vi "Update Indicators.vi"(8 "error in (no error)":errorcluster, 11 "Bioreactor in":refnum<class "Bioreactor.lvclass">) -> (0 "error out":errorcluster, 3 "Bioreactor out":refnum<class "Bioreactor.lvclass">)   [LabVIEW 2013, in "Bioreactor.lvlib" / "Bioreactor.lvclass"]
uses:
  Bioreactor.lvclass
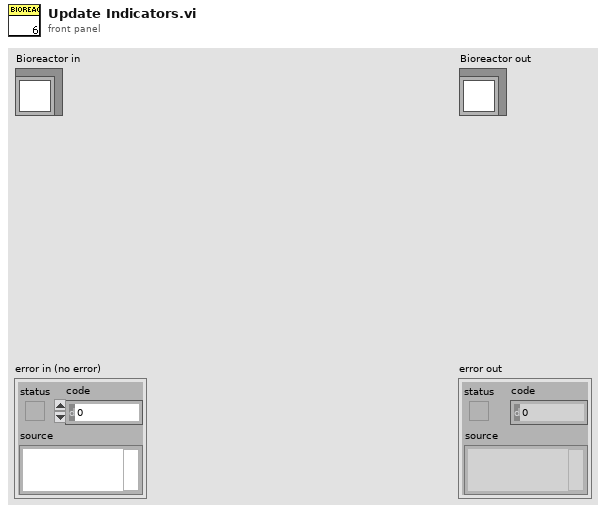
[diagram p1: front panel]
types:
  T1 = cluster{"output array":dbl[], "output array":dbl[]}
  T2 = cluster{"output array":dbl[], "output array":dbl[]}[]
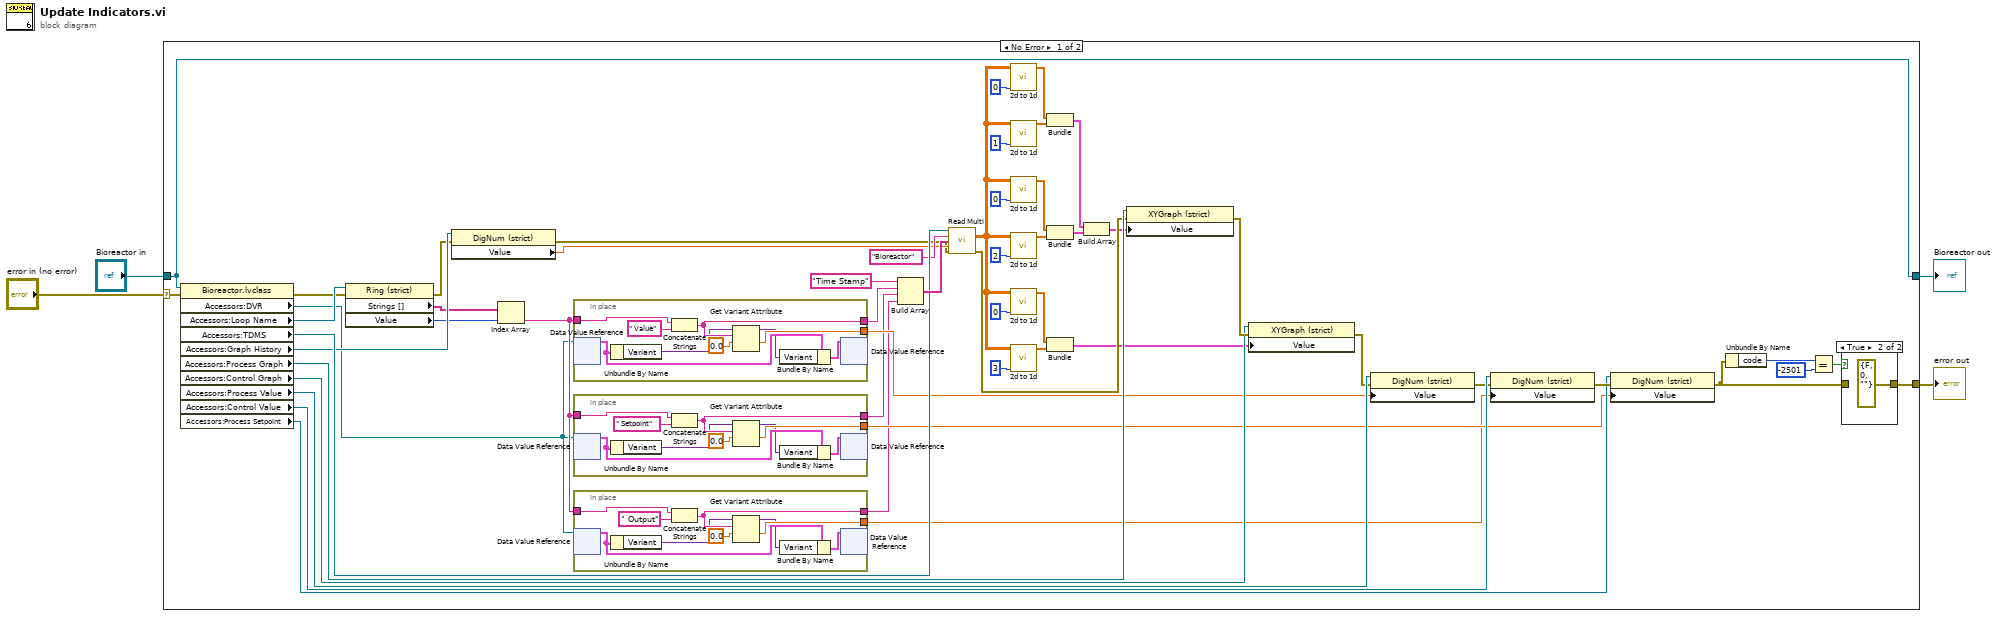
[diagram p0: block diagram]
diagram:
  n1 = case shown="No Error" "error in (no error)" {
    selector: "error in (no error)" -> [w54 w89]
    tunnel: [w18 w89] -> w3
    tunnel: [w58 w88] -> w1
    tunnel: "Bioreactor in" -> [w58 w88]
    frame No Error {
      n2 = property class="Bioreactor.lvclass"(reference=w58, error in=w54) -> (error out=w53:errorcluster, "Accessors:DVR"=w5:refnum<data-value>, "Accessors:Loop Name"=w55:refnum<vi>, "Accessors:TDMS"=w48:refnum<k34>, "Accessors:Graph History"=w37:refnum<vi>, "Accessors:Process Graph"=w35:refnum<vi>, "Accessors:Control Graph"=w36:refnum<vi>, "Accessors:Process Value"=w57:refnum<vi>, "Accessors:Control Value"=w56:refnum<vi>, "Accessors:Process Setpoint"=w50:refnum<vi>)  [unwired: 1 out]
      n3 = property class="Ring (strict)"(reference=w55, error in=w53) -> (error out=w17:errorcluster, "Strings []"=w15:string[], "Value"=w16:u16)  [unwired: 1 out]
      n4 = property class="DigNum (strict)"(reference=w37, error in=w17) -> (error out=w13:errorcluster, "Value"=w14:dbl)  [unwired: 1 out]
      n5 = Index Array(array=w15, index=w16) -> (element=w6:string)
      n6 = in-place {
        in-place-border: w6 -> [w67]
        in-place-border: [w64] -> w12
        in-place-border: [w63] -> w7
        n7 = in-place-dvr #1(w5) -> (w62:cluster{"Array":string[], "Variant":variant})  [unwired: 1 out]
        n8 = Unbundle By Name(w62) -> ("Variant"=w61:variant)
        n9 = Concatenate Strings(w67, " Value" ("string")) -> (w63:string)
        n10 = Get Variant Attribute(Variant=w61, name=w63, default value (empty Variant)=0.0 ("Value")) -> (duplicate Variant=w60:variant, value=w64:dbl)  [unwired: 1 in, 2 out]
        n11 = Bundle By Name(cluster=w62, "Variant"=w60) -> (w59:cluster{"Array":string[], "Variant":variant})
        n12 = in-place-dvr #1(w59) -> ()  [unwired: 2 out]
      }
      n13 = in-place {
        in-place-border: w6 -> [w85]
        in-place-border: [w84] -> w11
        in-place-border: [w81] -> w9
        n14 = in-place-dvr #2(w5) -> (w80:cluster{"Array":string[], "Variant":variant})  [unwired: 1 out]
        n15 = Unbundle By Name(w80) -> ("Variant"=w79:variant)
        n16 = Concatenate Strings(w85, " Setpoint" ("string")) -> (w81:string)
        n17 = Get Variant Attribute(Variant=w79, name=w81, default value (empty Variant)=0.0 ("Value")) -> (duplicate Variant=w78:variant, value=w84:dbl)  [unwired: 1 in, 2 out]
        n18 = Bundle By Name(cluster=w80, "Variant"=w78) -> (w77:cluster{"Array":string[], "Variant":variant})
        n19 = in-place-dvr #2(w77) -> ()  [unwired: 2 out]
      }
      n20 = in-place {
        in-place-border: w6 -> [w76]
        in-place-border: [w75] -> w10
        in-place-border: [w72] -> w8
        n21 = in-place-dvr #3(w5) -> (w71:cluster{"Array":string[], "Variant":variant})  [unwired: 1 out]
        n22 = Unbundle By Name(w71) -> ("Variant"=w70:variant)
        n23 = Concatenate Strings(w76, " Output" ("string")) -> (w72:string)
        n24 = Get Variant Attribute(Variant=w70, name=w72, default value (empty Variant)=0.0 ("Value")) -> (duplicate Variant=w69:variant, value=w75:dbl)  [unwired: 1 in, 2 out]
        n25 = Bundle By Name(cluster=w71, "Variant"=w69) -> (w68:cluster{"Array":string[], "Variant":variant})
        n26 = in-place-dvr #3(w68) -> ()  [unwired: 2 out]
      }
      n27 = Build Array("Time Stamp" ("string"), w7, w9, w8) -> (w49:string[])
      n28 = call "Read Multi.vi"("tdms file in"=w48, "group"="Bioreactor", "Channel"=w49, "Numeric"=w14, "error in (no error)"=w13) -> ("Array"=w40:dbl[][], "error out"=w34:errorcluster)  [unwired: 7 in, 2 out]
      n29 = call "2d to 1d.vi"("index"=0, "array"=w40) -> ("output array"=w30:dbl[])  [unwired: 9 in]
      n30 = call "2d to 1d.vi"("index"=1, "array"=w40) -> ("output array"=w29:dbl[])  [unwired: 9 in]
      n31 = call "2d to 1d.vi"("index"=0, "array"=w40) -> ("output array"=w32:dbl[])  [unwired: 9 in]
      n32 = call "2d to 1d.vi"("index"=2, "array"=w40) -> ("output array"=w31:dbl[])  [unwired: 9 in]
      n33 = call "2d to 1d.vi"("index"=0, "array"=w40) -> ("output array"=w25:dbl[])  [unwired: 9 in]
      n34 = call "2d to 1d.vi"("index"=3, "array"=w40) -> ("output array"=w24:dbl[])  [unwired: 9 in]
      n35 = Bundle("output array"=w30, "output array"=w29) -> (w28:T1)  [unwired: 1 in]
      n36 = Bundle("output array"=w32, "output array"=w31) -> (w27:T1)  [unwired: 1 in]
      n37 = Bundle("output array"=w25, "output array"=w24) -> (w23:T1)  [unwired: 1 in]
      n38 = Build Array(w28, w27) -> (w26:T2)
      n39 = property class="XYGraph (strict)"(reference=w35, error in=w34, "Value"=w26) -> (error out=w39:errorcluster)  [unwired: 1 out]
      n40 = property class="XYGraph (strict)"(reference=w36, error in=w39, "Value"=w23) -> (error out=w38:errorcluster)  [unwired: 1 out]
      n41 = property class="DigNum (strict)"(reference=w57, error in=w38, "Value"=w12) -> (error out=w52:errorcluster)  [unwired: 1 out]
      n42 = property class="DigNum (strict)"(reference=w56, error in=w52, "Value"=w10) -> (error out=w51:errorcluster)  [unwired: 1 out]
      n43 = property class="DigNum (strict)"(reference=w50, error in=w51, "Value"=w11) -> (error out=w19:errorcluster)  [unwired: 1 out]
      n44 = Unbundle By Name(w19) -> ("code"=w22:i32)
      n45 = Equal?(x=w22, y=-2501) -> (x = y?=w20:bool)
      n46 = case shown="True" w20 {
        tunnel: w19 -> [w86 _]
        tunnel: [w86 errorcluster {"status"=FALSE, "code"=0, "source"=""} ("error constant")] -> w18
        frame False {
        }
        frame True {
        }
      }
    }
    frame Error {
    }
  }
  "error out" <- w3
  "Bioreactor out" <- w1
